vi "Setting_target_temp.vi"() -> ()   [LabVIEW 2016]
uses:
  Thermal_type.vi
panel:
  in  "User Target temp":dbl
  out "Type Transducer":string
  in  "취소 버튼":bool
  in  "Initial PRF":dbl=2000.0 format="%.2f"
  out "Setting target temp":dbl[](array[numeric])
  in  "Target temperature raw data":dbl[][](array[numeric])=[[35.0, 35.0, 35.0, 35.0, 35.0, 35.0, 35.0, 35.0, 35.0, 35.0], [26.0, 28.0, 30.0, 32.0, 34.0, 35.0, 35.0, 35.0, 35.0, 35.0], [29.0, 31.0, 33.0, 35.0, 36.0, 37.0, 37.0, 37.0, 37.0, 37.0]]
  in  "확인 버튼":bool
  in  "Setting Target Temperature":i8(slide) scale=0.0..3.0
  out "Setting Target Temperature Data":dbl[](graph)
  # "PID Control for PRF"
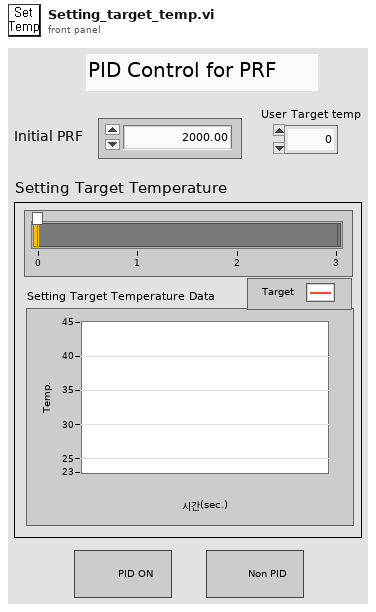
[diagram p1: front panel]
types:
  T1 = enum8{"Enabled", "Disabled", "Disabled and Grayed Out"}
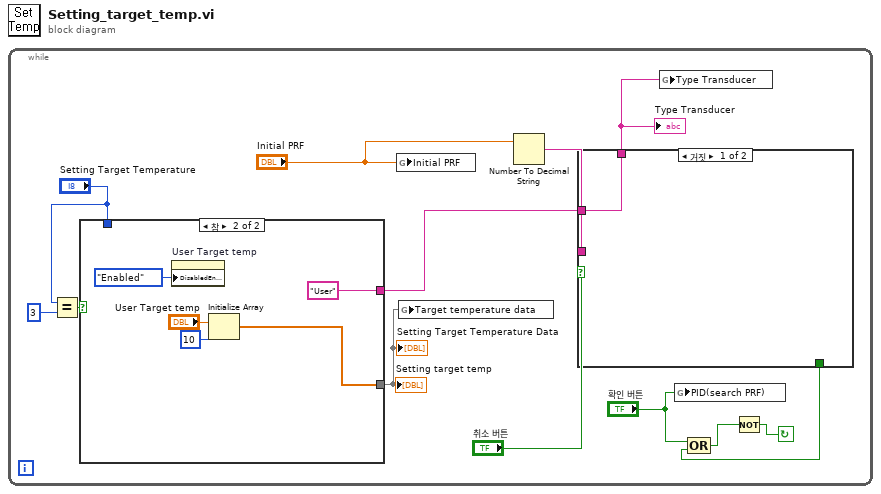
[diagram p0: block diagram]
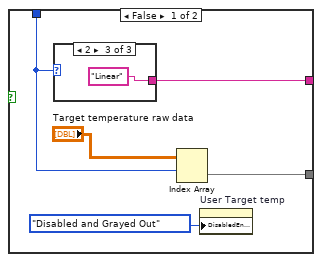
[diagram p2: hidden frame]
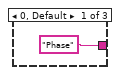
[diagram p3: hidden frame]
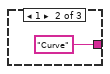
[diagram p4: hidden frame]
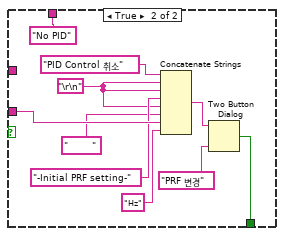
[diagram p5: hidden frame]
diagram:
  n1 = while {
    stop <- w13 continue-if-true
    n2 = Equal?(x="Setting Target Temperature", y=i8 3) -> (x = y?=w5:bool)
    n3 = case shown="참" w5 {
      tunnel: [w18 w23] -> w12
      tunnel: "Setting Target Temperature" -> [w16 _]
      tunnel: [w15 "User"] -> w2
      frame False {
        n4 = case shown="2" w16 {
          tunnel: ["Phase" "Curve" "Linear"] -> w15
          frame 0, Default {
          }
          frame 1 {
          }
          frame 2 {
          }
        }
        n5 = Index Array(array="Target temperature raw data", index (row)=w16) -> (element=w18:dbl[])  [unwired: 1 in]
        n6 = property on="User Target temp" class="DigNum (엄격한)"("DisabledEnum"=T1."Disabled and Grayed Out" ("비활성화")) -> ()  [unwired: 2 in, 2 out]
      }
      frame True {
        n7 = property on="User Target temp" class="DigNum (엄격한)"("DisabledEnum"=T1."Enabled" ("비활성화")) -> ()  [unwired: 2 in, 2 out]
        n8 = Initialize Array("User Target temp", 10 ("차원 크기")) -> (w23:dbl[])
      }
    }
    "Setting Target Temperature Data" <- w12
    "Setting target temp" <- w12
    n9 = global write "Thermal_type.vi" "Initial PRF"("Initial PRF") -> ()
    n10 = global write "Thermal_type.vi" "Target temperature data"(w12) -> ()
    n11 = Number To Decimal String(number="Initial PRF") -> (decimal integer string=w8:string)  [unwired: 1 in]
    n12 = case shown="거짓" "취소 버튼" {
      tunnel: w8 -> [_ w33]
      tunnel: [_ w35] -> w6
      tunnel: [w27 "No PID"] -> w1
      tunnel: w2 -> [w27 _]
      frame False {
      }
      frame True {
        w31 = "\r\n"
        n13 = Concatenate Strings("PID Control 취소" ("문자열"), w31, w31, "-Initial PRF setting-" ("문자열"), w31, "        ", w33, "Hz" ("문자열")) -> (w36:string)
        n14 = Two Button Dialog(message=w36, 1:"PRF 변경" ("거짓 버튼 이름(\"취소\")")) -> (T button?=w35:bool)  [unwired: 1 in]
      }
    }
    "Type Transducer" <- w1
    n15 = global write "Thermal_type.vi" "Type Transducer"(w1) -> ()
    n16 = global write "Thermal_type.vi" "PID(search PRF)"("확인 버튼") -> ()
    n17 = Compound Arithmetic op=OR("확인 버튼", w6) -> (w10:bool)
    n18 = Not(x=w10) -> (.not. x?=w13:bool)
  }
